vi "_DServerRequestTypeToString.vi"(1 "request type":T1=enum."UNKNOWN_REQUEST") -> (0 "request type str":string="UNKNOWN_REQ")   [LabVIEW 2014, in "tango.lvlib"]
uses:
  tango.lvlib
  Client Request Handling/Typedefs/_DServerClientRequestType.ctl
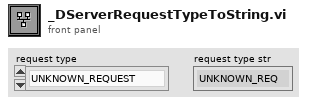
[diagram p1: front panel]
types:
  T1 = typedef "tango.lvlib/_DServerClientRequestType.ctl" = enum16{"EXEC_CMD", "READ_ATTR", "WRITE_ATTR", "UNKNOWN_REQUEST"}
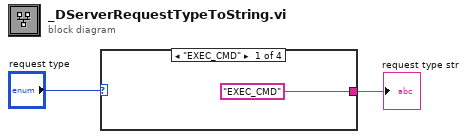
[diagram p0: block diagram]
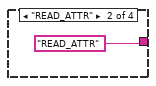
[diagram p2: hidden frame]
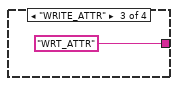
[diagram p3: hidden frame]
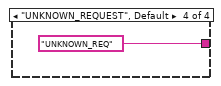
[diagram p4: hidden frame]
diagram:
  n1 = case shown="\"EXEC_CMD\"" "request type" {
    tunnel: ["EXEC_CMD" "READ_ATTR" "WRT_ATTR" "UNKNOWN_REQ"] -> w1
    frame "EXEC_CMD" {
    }
    frame "READ_ATTR" {
    }
    frame "WRITE_ATTR" {
    }
    frame "UNKNOWN_REQUEST", Default {
    }
  }
  "request type str" <- w1
